vi "RSZVB Set Trace Smoothing.vi"(7 "Aperture (1.0 %)":dbl=1.0 format="%^.3e", 8 "error in (no error)":errorcluster {"code" format="%.0x"}, 9 "Smoothing (F: Off)":bool, 10 "Channel (Trace) (1)":i32=1, 11 "VISA session":refnum<visa-resource-name>) -> (0 "error out":errorcluster {"code" format="%.0x"}, 3 "dup VISA session":refnum<visa-resource-name>)   [LabVIEW 2011]
doc: "This VI activates the smoothing VI for the active trace, which may be a data or a memory trace. With active smoothing VI, each measurement point is replaced by the arithmetic mean value of all measurement points located in a symmetric interval centered on the stimulus value. The width of the smoothing interval is referred to as the Smoothing Apertureand can be adjusted according to the properties of the trace. \n\nRemote-control command(s):\nCALCulate<Ch/Tr>:SMOothing[:STATe] <Boolean>\nCALCulate<Ch/Tr>:SMOothing:APERture <numeric_value>"
panel:
  # "On\nOff"
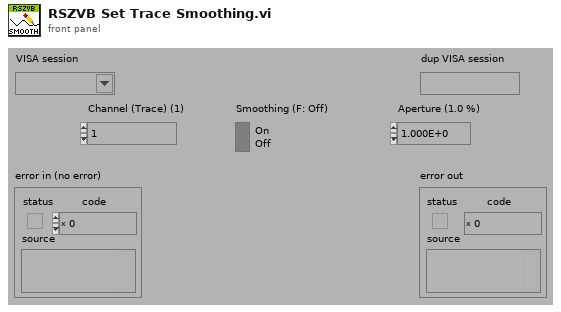
[diagram p1: front panel]
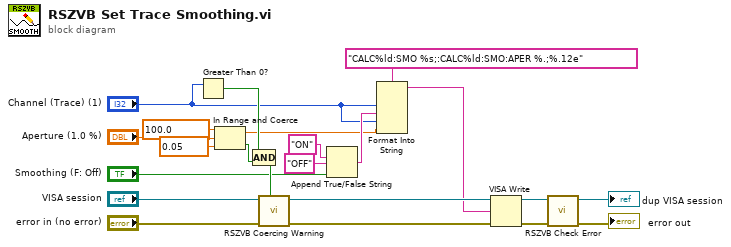
[diagram p0: block diagram]
diagram:
  n1 = Greater Than 0?(x="Channel (Trace) (1)") -> (x > 0?=w15:bool)
  n2 = In Range and Coerce(upper limit=100.0, x="Aperture (1.0 %)", lower limit=0.05) -> (coerced(x)=w1:dbl, In Range?=w8:bool)
  n3 = Compound Arithmetic op=AND(w15, w8) -> (w14:bool)
  n4 = call "RSZVB Coercing Warning.vi"("In Range?"=w14, "error in (no error)"="error in (no error)", "VISA session"="VISA session") -> ("error out"=w21:errorcluster, "dup VISA session"=w22:refnum<visa-resource-name>)  [unwired: 7 in]
  n5 = Append True/False String(1:"Smoothing (F: Off)", 2:"OFF", 3:"ON") -> (0:w6:string)  [unwired: 1 in]
  n6 = Format Into String(format string="CALC%ld:SMO %s;:CALC%ld:SMO:APER %.;%.12e", "Channel (Trace) (1)", w6, "Channel (Trace) (1)", w1) -> (resulting string=w3:string)  [unwired: 2 in, 1 out]
  n7 = VISA Write(VISA resource name=w22, write buffer=w3, error in (no error)=w21) -> (VISA resource name out=w19:refnum<visa-resource-name>, error out=w20:errorcluster)  [unwired: 1 out]
  n8 = call "RSZVB Check Error.vi"("error in (no error)"=w20, "VISA session"=w19) -> ("error out"=→"error out":errorcluster, "dup VISA session"=→"dup VISA session":refnum<visa-resource-name>)  [unwired: 8 in]
